vi "Config Daq.vi"(3 "Device":u16(ring) items=["Dev6", "Dev10", "Dev11"]) -> (0 "AI voltage":dbl[](array[numeric]), 1 "samples per read out":i32=10 min=1 max=25 step=1, 2 "Data rate out (hz)":dbl=500.0 min=1.0 max=2500.0 step=1.0 format="%#.0f", 4 "AI Channels":string[](array[string]), 5 "Device Name":string, 6 "Buffer out":i32)   [LabVIEW 2019]
uses:
  AI voltages.ctl
  Calibration and Function folders.ctl
  DAQ configuration/Sensor buffer command.ctl
  <vilib>/Utility/config.llb/Write Key (Double).vi
  <vilib>/Utility/config.llb/Write Key (I32).vi
  <vilib>/Utility/config.llb/Write Key (String).vi
  <vilib>/Utility/config.llb/NI_LVConfig.lvlib
panel:
  in  "Max Voltage for data type":T1
  out "Seconds stored in buffer":dbl
  in  "Buffer":i32
  out "Devices":string[](array[string])
  in  "Cancel Button":bool
  in  "OK Button":bool
  in  "Max Voltage":T1[](array[typedef])=[enum."1 V", enum."1 V", enum."1 V", enum."1 V"]
  out "error out":errorcluster
  in  "error in":errorcluster
  in  "Data rate (hz)":dbl=500.0 min=1.0 max=2500.0 step=1.0 format="%#.0f"
  in  "samples per read":i32=10 min=1 max=25 step=1
  # "Select from the list of available devices"
  # "Set the maximum voltage for each channel. Use the lowest voltage that is greater than the maximum voltage produced by your sensors."
  # "Use spacebar to access these data rates and buffer size if needed.  Data rate is at the data acquisition board. Samples per read results in immediate averaging before storage in the buffer. The buffer is used by ProCoDA to create longer term averages for process control"
  # "The maximum data rate is 2500 hz."
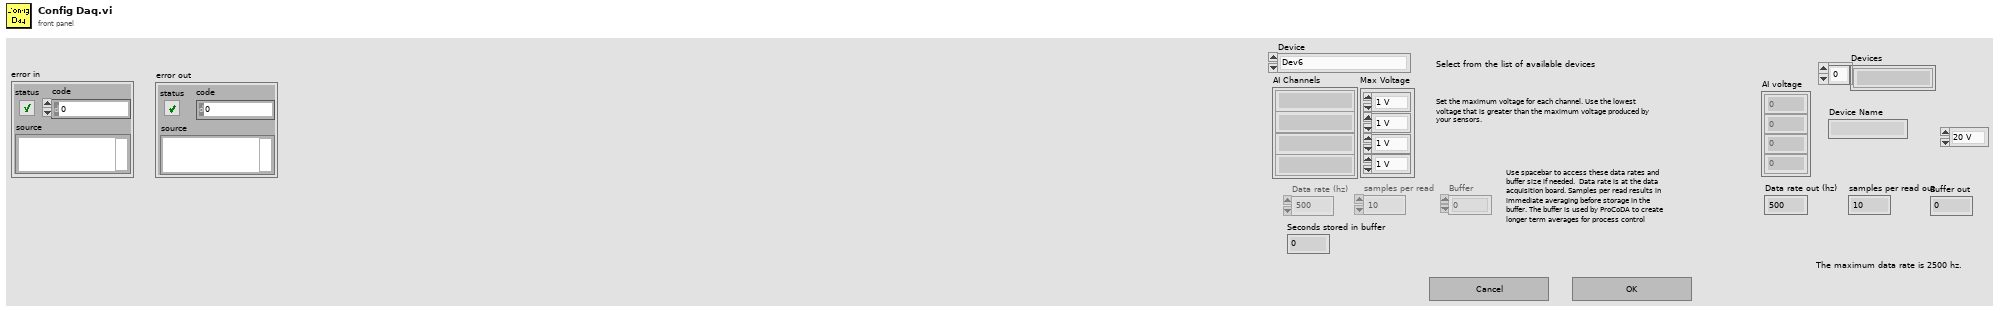
[diagram p1: front panel]
types:
  T1 = typedef "AI voltages.ctl" = enum16{"20 V", "10 V", "5 V", "4 V", "2.5 V", "2 V", "1.25 V", "1 V"}
  T2 = typedef "Sensor buffer command.ctl" = enum16{"read average", "read recent", "read all", "write", "set buffer size", "Read channel config", "Write channel config", "clear"}
  T3 = typedef "Calibration and Function folders.ctl" = enum16{"Sensors", "Functions", "Config File", "PublicAppFolder", "New ini File", "Set Config File", "Delete ini File"}
  T4 = enum8{"Enabled", "Disabled", "Disabled and Grayed Out"}
  T5 = typedef "NI_LVConfig.lvlib/Config Data RefNum.ctl" = refnum<k1>
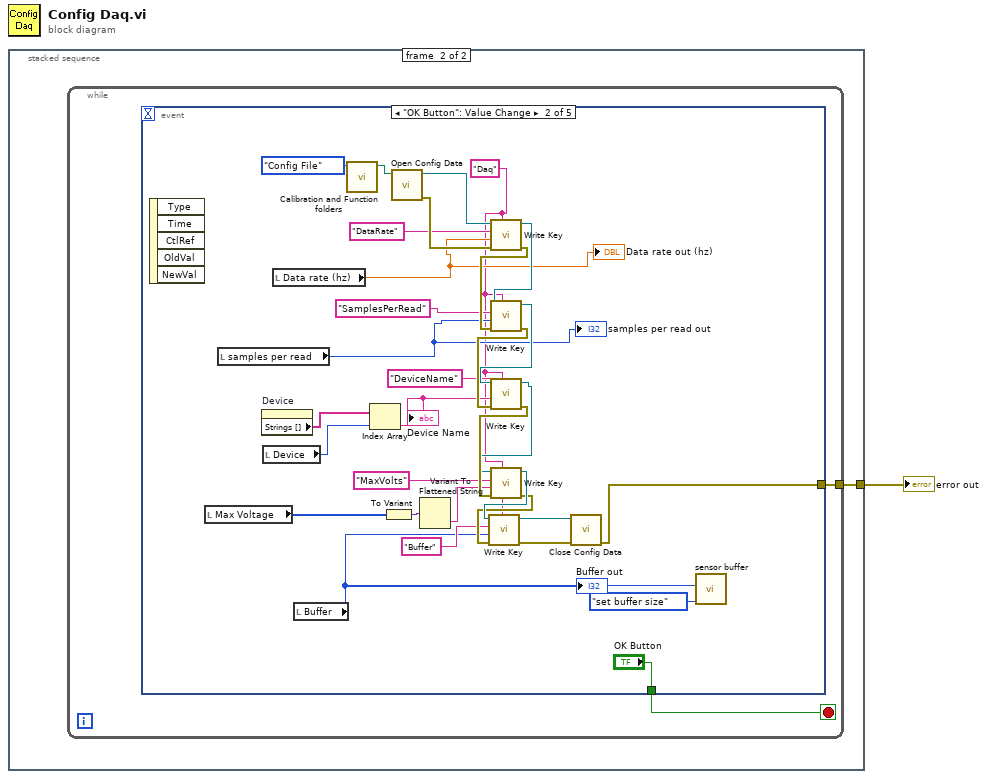
[diagram p0: block diagram]
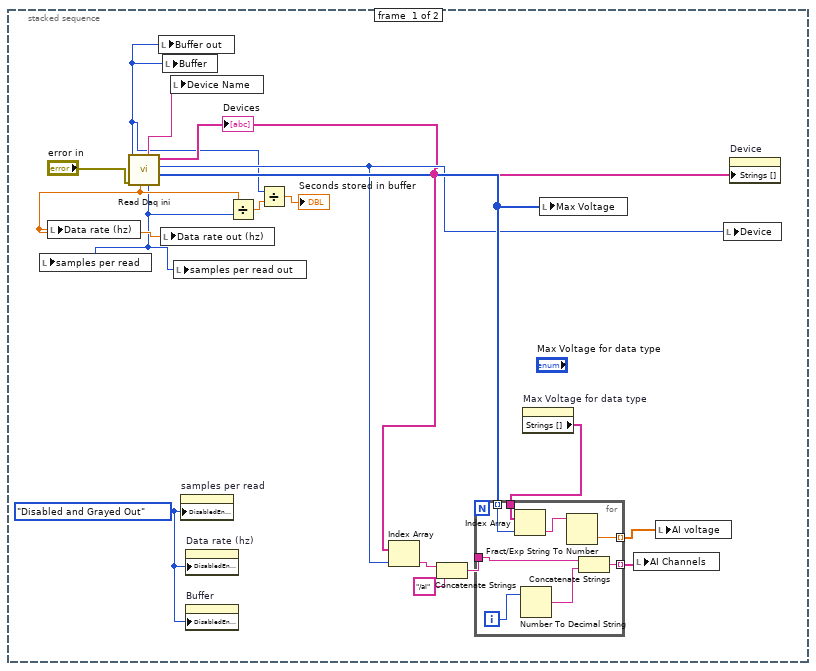
[diagram p2: hidden frame]
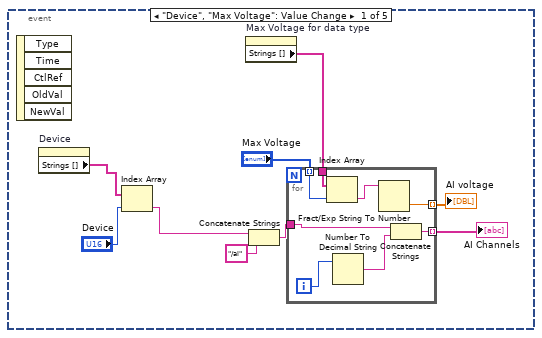
[diagram p3: hidden frame]
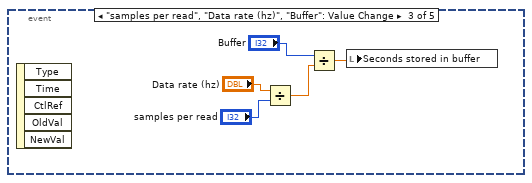
[diagram p4: hidden frame]
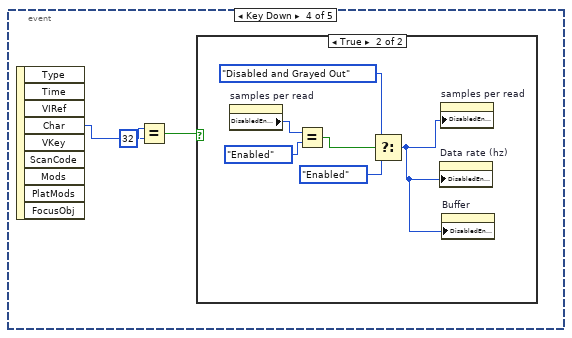
[diagram p5: hidden frame]
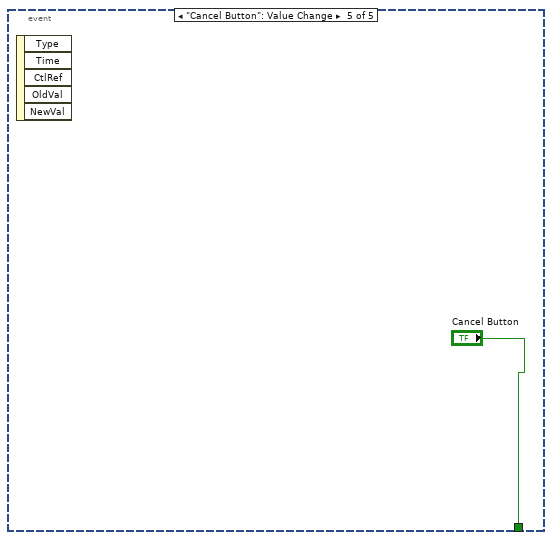
[diagram p7: hidden frame]
diagram:
  n1 = stacked-sequence {
    tunnel: [_ w27] -> w1
    frame #0 {
      w8 = T4."Disabled and Grayed Out" ("Disabled")
      n2 = call "Read Daq ini.vi"("error in"="error in") -> ("Max Voltage"=w13:T1[], "Device"=w11:u16, "Devices"=w10:string[], "samples per read"=w6:i32, "DeviceName"=w9:string, "Data rate (hz)"=w7:dbl, "Buffer"=w4:i32)  [unwired: 2 in, 2 out]
      "Devices" <- w10
      n3 = local write "samples per read"(w6) -> ()
      n4 = local write "Data rate (hz)"(w7) -> ()
      n5 = local write "Buffer out"(w4) -> ()
      n6 = local write "Data rate out (hz)"(w7) -> ()
      n7 = local write "Buffer"(w4) -> ()
      n8 = local write "Device Name"(w9) -> ()
      n9 = local write "samples per read out"(w6) -> ()
      n10 = property on="samples per read" class="DigNum (strict)"("DisabledEnum"=w8) -> ()  [unwired: 2 in, 2 out]
      n11 = property on="Data rate (hz)" class="DigNum (strict)"("DisabledEnum"=w8) -> ()  [unwired: 2 in, 2 out]
      n12 = property on="Buffer" class="DigNum (strict)"("DisabledEnum"=w8) -> ()  [unwired: 2 in, 2 out]
      n13 = Divide(x=w7, y=w6) -> (x/y=w5:dbl)
      n14 = Divide(x=w4, y=w5) -> (x/y=→"Seconds stored in buffer":dbl)
      n15 = Index Array(array=w10, index=w11) -> (element=w12:string)
      n16 = Concatenate Strings(w12, "/ai") -> (w16:string)
      n17 = property on="Max Voltage for data type" class="Enum (strict)"() -> ("Strings []"=w2:string[])  [unwired: 2 in, 2 out]
      n18 = for {
        tunnel: w16 -> [w26]
        tunnel: [w23] -> w18 mode=indexing
        tunnel: w2 -> [w22]
        tunnel: w13 -> [w21] mode=indexing
        tunnel: [w19] -> w17 mode=indexing
        i -> [w25]
        n19 = Index Array(array=w22, index=w21) -> (element=w20:string)
        n20 = Number To Decimal String(number=w25) -> (decimal integer string=w24:string)  [unwired: 1 in]
        n21 = Fract/Exp String To Number(string=w20) -> (number=w19:dbl)  [unwired: 3 in, 1 out]
        n22 = Concatenate Strings(w26, w24) -> (w23:string)
      }
      n23 = local write "Max Voltage"(w13) -> ()
      n24 = local write "AI Channels"(w18) -> ()
      n25 = local write "AI voltage"(w17) -> ()
      n26 = local write "Device"(w11) -> ()
      n27 = property on="Device" class="Ring (strict)"("Strings []"=w10) -> ()  [unwired: 2 in, 2 out]
    }
    frame #1 {
      n28 = while {
        tunnel: [w28] -> w27
        stop <- w29 stop-if-true
        n29 = event shown="[1] \"OK Button\": Value Change" {
          selector: _ -> [_ _ _ _ _]
          dyn-events: _ -> [_ _ _ _ _]
          timeout: _ -> [_ _ _ _ _]
          tunnel: [_ "OK Button" _ _ "Cancel Button"] -> w29
          tunnel: [_ w59 _ _ _] -> w28
          event "Device", "Max Voltage": Value Change {
            n30 = event-data() -> ()  [unwired: 1 in, 5 out]
            n31 = property on="Device" class="Ring (strict)"() -> ("Strings []"=w38:string[])  [unwired: 2 in, 2 out]
            n32 = Index Array(array=w38, index="Device") -> (element=w31:string)
            n33 = property on="Max Voltage for data type" class="Enum (strict)"() -> ("Strings []"=w30:string[])  [unwired: 2 in, 2 out]
            n34 = Concatenate Strings(w31, "/ai") -> (w35:string)
            n35 = for {
              tunnel: w35 -> [w46]
              tunnel: [w43] -> w34 mode=indexing
              tunnel: w30 -> [w42]
              tunnel: "Max Voltage" -> [w41] mode=indexing
              tunnel: [w39] -> w32 mode=indexing
              i -> [w45]
              n36 = Index Array(array=w42, index=w41) -> (element=w40:string)
              n37 = Number To Decimal String(number=w45) -> (decimal integer string=w44:string)  [unwired: 1 in]
              n38 = Fract/Exp String To Number(string=w40) -> (number=w39:dbl)  [unwired: 3 in, 1 out]
              n39 = Concatenate Strings(w46, w44) -> (w43:string)
            }
            "AI Channels" <- w34
            "AI voltage" <- w32
          }
          event "OK Button": Value Change {
            w51 = "Daq" ("section")
            n40 = event-data() -> ()  [unwired: 1 in, 5 out]
            n41 = local read "Max Voltage"() -> (w61:T1[])
            n42 = local read "samples per read"() -> (w52:i32)
            "samples per read out" <- w52
            n43 = property on="Device" class="Ring (strict)"() -> ("Strings []"=w65:string[])  [unwired: 2 in, 2 out]
            n44 = local read "Device"() -> (w64:u16)
            n45 = local read "Data rate (hz)"() -> (w53:dbl)
            "Data rate out (hz)" <- w53
            n46 = local read "Buffer"() -> (w49:i32)
            "Buffer out" <- w49
            n47 = call "Calibration and Function folders.vi"("Folder"=Calibration_and_Function_folders."Config File") -> ("Selected Folder"=w48:path)  [unwired: 9 in, 1 out]
            n48 = Index Array(array=w65, index=w64) -> (element=w63:string)
            "Device Name" <- w63
            n49 = To Variant(anything=w61) -> (Variant=w62:variant)
            n50 = call <vilib>:"Open Config Data.vi"("configuration file path"=w48) -> ("error out"=w77:errorcluster, "refnum"=w73:T5)  [unwired: 8 in, 1 out]
            n51 = Variant To Flattened String(Variant=w62) -> (data string=w60:string)  [unwired: 1 out]
            n52 = call-poly <vilib>:"Write Key.vi"("section"=w51, "error in (no error)"=w77, "value"=w53, "key"="DataRate", "refnum"=w73) -> ("error out"=w76:errorcluster, "refnum out"=w72:T5)  [unwired: 4 in, 1 out]
            n53 = call-poly <vilib>:"Write Key.vi"("section"=w51, "error in (no error)"=w76, "value"=w52, "key"="SamplesPerRead", "refnum"=w72) -> ("error out"=w75:errorcluster, "refnum out"=w71:T5)  [unwired: 4 in, 1 out]
            n54 = call-poly <vilib>:"Write Key.vi"("section"=w51, "error in (no error)"=w75, "value"=w63, "key"="DeviceName", "refnum"=w71) -> ("error out"=w74:errorcluster, "refnum out"=w70:T5)  [unwired: 4 in, 1 out]
            n55 = call-poly <vilib>:"Write Key.vi"("section"=w51, "error in (no error)"=w74, "value"=w60, "key"="MaxVolts", "refnum"=w70) -> ("error out"=w57:errorcluster, "refnum out"=w58:T5)  [unwired: 4 in, 1 out]
            n56 = call-poly <vilib>:"Write Key.vi"("section"=w51, "error in (no error)"=w57, "value"=w49, "key"="Buffer", "refnum"=w58) -> ("error out"=w54:errorcluster, "refnum out"=w55:T5)  [unwired: 4 in, 1 out]
            n57 = call <vilib>:"Close Config Data.vi"("error in (no error)"=w54, "refnum"=w55) -> ("error out"=w59:errorcluster)  [unwired: 8 in, 1 out]
            n58 = call "sensor buffer.vi"("command"=Sensor_buffer_command."set buffer size", "max array size"=w49) -> ()  [unwired: 5 in, 5 out]
          }
          event "samples per read", "Data rate (hz)", "Buffer": Value Change {
            n59 = event-data() -> ()  [unwired: 1 in, 5 out]
            n60 = Divide(x="Data rate (hz)", y="samples per read") -> (x/y=w80:dbl)
            n61 = Divide(x="Buffer", y=w80) -> (x/y=w79:dbl)
            n62 = local write "Seconds stored in buffer"(w79) -> ()
          }
          event Key Down {
            n63 = event-data() -> ("Char"=w86:i16)  [unwired: 1 in, 8 out]
            n64 = Equal?(x=w86, y=i16 32) -> (x = y?=w84:bool)
            n65 = case shown="True" w84 {
              frame False {
              }
              frame True {
                n66 = property on="samples per read" class="DigNum (strict)"() -> ("DisabledEnum"=w92:T4)  [unwired: 2 in, 2 out]
                n67 = Equal?(x=w92, y=T4."Enabled" ("Disabled")) -> (x = y?=w90:bool)
                n68 = Select(t=T4."Disabled and Grayed Out" ("Disabled"), s=w90, f=T4."Enabled" ("Disabled")) -> (s? t:f=w87:T4)
                n69 = property on="Data rate (hz)" class="DigNum (strict)"("DisabledEnum"=w87) -> ()  [unwired: 2 in, 2 out]
                n70 = property on="samples per read" class="DigNum (strict)"("DisabledEnum"=w87) -> ()  [unwired: 2 in, 2 out]
                n71 = property on="Buffer" class="DigNum (strict)"("DisabledEnum"=w87) -> ()  [unwired: 2 in, 2 out]
              }
            }
          }
          event "Cancel Button": Value Change {
            n72 = event-data() -> ()  [unwired: 1 in, 5 out]
          }
        }
      }
    }
  }
  "error out" <- w1
